vi "MPExxx_err.vi"(1 "error in (no error)":errorcluster) -> (0 "error out":errorcluster)   [LabVIEW 2017]
doc: "This form removes the termination character found warning."
panel:
  # "MAGNA-POWER"
  # "Electronics"
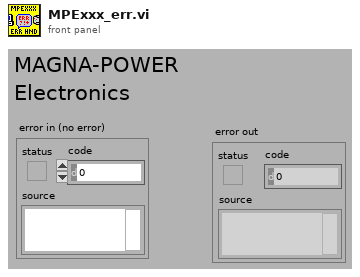
[diagram p1: front panel]
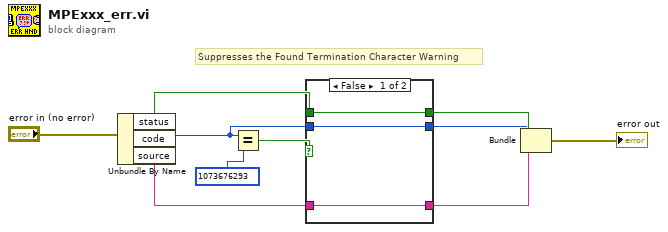
[diagram p0: block diagram]
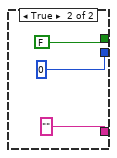
[diagram p2: hidden frame]
diagram:
  # "Suppresses the Found Termination Character Warning"
  n1 = Unbundle By Name("error in (no error)") -> ("status"=w10:bool, "code"=w7:i32, "source"=w6:string)
  n2 = Equal?(x=w7, y=1073676293) -> (x = y?=w9:bool)
  n3 = case shown="False" w9 {
    tunnel: w10 -> [w13 _]
    tunnel: w7 -> [w12 _]
    tunnel: [w13 FALSE] -> w5
    tunnel: w6 -> [w11 _]
    tunnel: [w12 0] -> w3
    tunnel: [w11 ""] -> w4
    frame False {
    }
    frame True {
    }
  }
  n4 = Bundle("status"=w5, "code"=w3, "source"=w4) -> (→"error out":errorcluster)  [unwired: 1 in]
